vi "KB-二维数组排序.vi"(10 "平均个数":i32=10, 11 "二维数组":dbl[][](array[numeric])) -> (3 "平均最高值":dbl)   [LabVIEW 2015]
panel:
  out "数组 2":dbl[](array[numeric])
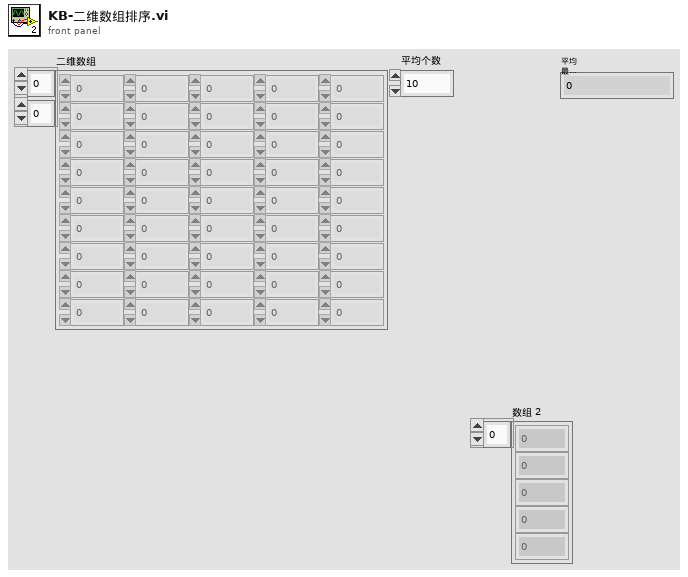
[diagram p1: front panel]
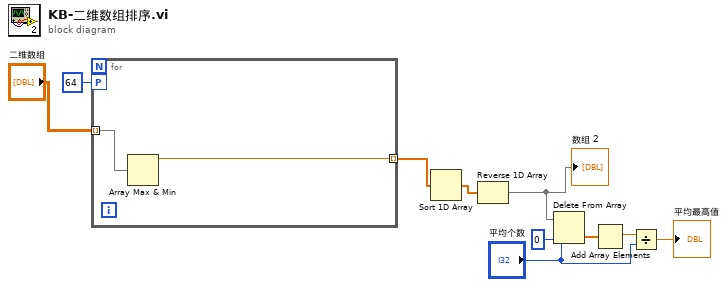
[diagram p0: block diagram]
diagram:
  n1 = for {
    tunnel: "二维数组" -> [w12] mode=indexing
    tunnel: [w11] -> w8 mode=indexing
    workers-P: 64 -> [_]
    n2 = Array Max & Min(array=w12) -> (max value=w11:dbl)  [unwired: 3 out]
  }
  n3 = Sort 1D Array(array=w8) -> (sorted array=w7:dbl[])
  n4 = Reverse 1D Array(array=w7) -> (reversed array=w6:dbl[])
  "数组 2" <- w6
  n5 = Delete From Array(array=w6, length="平均个数", index=0 ("索引")) -> (deleted portion=w4:dbl[])  [unwired: 1 out]
  n6 = Add Array Elements(numeric array=w4) -> (sum=w3:dbl)
  n7 = Divide(x=w3, y="平均个数") -> (x/y=→"平均最高值":dbl)
